vi "Dashboard Main.vi"() -> ()   [LabVIEW 2017]
uses:
  <vilib>/Utility/miscctls.llb/LVRowAndColumnTypeDef.ctl
  <vilib>/event_ctls.llb/eventvkey.ctl
  <vilib>/Rock Robotics/Network Tables/NT Read Numeric Array.vi
  <vilib>/Rock Robotics/Network Tables/NT Read Boolean.vi
  <vilib>/Rock Robotics/WPI/Dashboard/WPI_DashboardLogging Global.vi
panel:
  in  "Camera Settings Right":T1={"Frame Rate"=30, "Compression"=30, "Size"=1, "DB Camera Config"=FALSE} {"Frame Rate" scale=1.0..30.0; "Compression" scale=100.0..-1.0; "Size" items=["640x480", "320x240", "160x120"]}
  in  "Camera Name Right":string(combo)="No Camera Selection"
  out "Camera Info":cluster{"Mbps LED":bool, "Mbps":dbl, "fps":dbl} {"fps" format="%#.1g"; "Mbps" format="%#.1g"}
  in  "Camera Settings":T1={"Frame Rate"=30, "Compression"=30, "Size"=1, "DB Camera Config"=FALSE} {"Frame Rate" scale=1.0..30.0; "Compression" scale=100.0..-1.0; "Size" items=["640x480", "320x240", "160x120"]}
  in  "TCP":refnum<k5>
  in  "Rec Mode":enum32{"Stop", "Record", "Playback"}(radio)
  out "Robot IP":string
  out "Image Message":string="Timeout in Camera Communications"
  in  "Dashboard Tab":T2(tab)
  in  "Select Auto":string(combo)="Select Autonomous ..."
  out "NT Connection":bool
  out "MotorChart R":cluster{"Numeric":dbl, "Numeric":dbl}(graph)
  out "MotorChart L":cluster{"Numeric":dbl, "Numeric":dbl}(graph)
  out "MotorSliders R":cluster{"MotorSlide1":dbl, "MotorSlide2":dbl} {"MotorSlide2" scale=-1.0..1.0 scale format="%#_2e"; "MotorSlide1" scale=-1.0..1.0 scale format="%#_2e"}
  out "MotorSliders L":cluster{"MotorSlide1":dbl, "MotorSlide2":dbl} {"MotorSlide2" scale=-1.0..1.0 scale format="%#_2e"; "MotorSlide1" scale=-1.0..1.0 scale format="%#_2e"}
  out "Gyro":dbl(knob) scale=0.0..360.0
  out "JS1 Z":dbl(slide) scale=-1.0..1.0 scale format="%#_2e"
  out "JS1 Graph":cluster{"X":dbl, "Y":dbl}[](graph)
  out "JS1 Buttons":T3
  out "JS2 Z":dbl(slide) scale=-1.0..1.0 scale format="%#_2e"
  out "JS2 Graph":cluster{"X":dbl, "Y":dbl}[](graph)
  out "JS2 Buttons":T3
  out "Mode":T4(ring)=enum."Auto Disabled"
  out "Camera Image Right":T5(plugin-control)
  in  "DB/String 9":string
  in  "DB/String 8":string
  in  "DB/String 7":string
  in  "DB/String 6":string
  in  "DB/String 5":string
  in  "DB/String 4":string
  in  "DB/String 3":string
  in  "DB/String 2":string
  in  "DB/String 1":string
  in  "DB/String 0":string
  in  "DB/Slider 0":dbl(slide) scale=0.0..5.0
  in  "DB/Slider 1":dbl(slide) scale=0.0..5.0
  in  "DB/Slider 2":dbl(slide) scale=0.0..5.0
  in  "DB/Slider 3":dbl(slide) scale=0.0..5.0
  out "DB/LED 3":bool
  out "DB/LED 2":bool
  out "DB/LED 1":bool
  out "DB/LED 0":bool
  in  "DB/Button 3":bool
  in  "DB/Button 2":bool
  in  "DB/Button 1":bool
  in  "DB/Button 0":bool caption="New Name"
  in  "Derrivative 2":dbl
  in  "Proportion 2":dbl
  in  "Integral 2":dbl
  in  "Derrivative":dbl
  in  "Integral":dbl
  in  "Proportion":dbl
  out "Lower Limit":bool
  out "Upper Limit":bool
  in  "Encoder distance":dbl
  in  "Test Slider":dbl(slide) scale=0.0..100.0 scale format="%#_3g"
  in  "On/Off":bool caption="Solenoid"
  in  "Test Name":u16(ring) items=["Select the test to run..."]
  in  "Test Tree":string(tree)
  in  "Motor":cluster{"Value":dbl, "Enable":bool} {"Value" scale=-1.0..1.0 scale format="%#_3g"}
  out "Progress":T6 {"Test Progress" scale=0.0..100.0}
  in  "Rev/Fwd":cluster{"Forward":bool, "Reverse":bool}
  in  "Test Ring":u16(ring) items=["Monochrome", "Color"]
  out "Cmd Status":string
  in  "Execute Command":bool
  in  "Command Params":string[][](table)
  in  "Command Selection":i32(listbox)
  in  "CheckList":i32(listbox)
  out "Tree":string(tree)
  out "Camera Image":T5(plugin-control)
  out "Background":bool
  in  "Camera Name":string(combo)="No Camera Selection"
  # "HW"
  # "HW"
  # "Joysticks"
  # "Drive Motors"
  # "Front"
  # "Right"
  # "Left"
  # "Back"
  # "Left Drive"
  # "Right (Follow)  Drive"
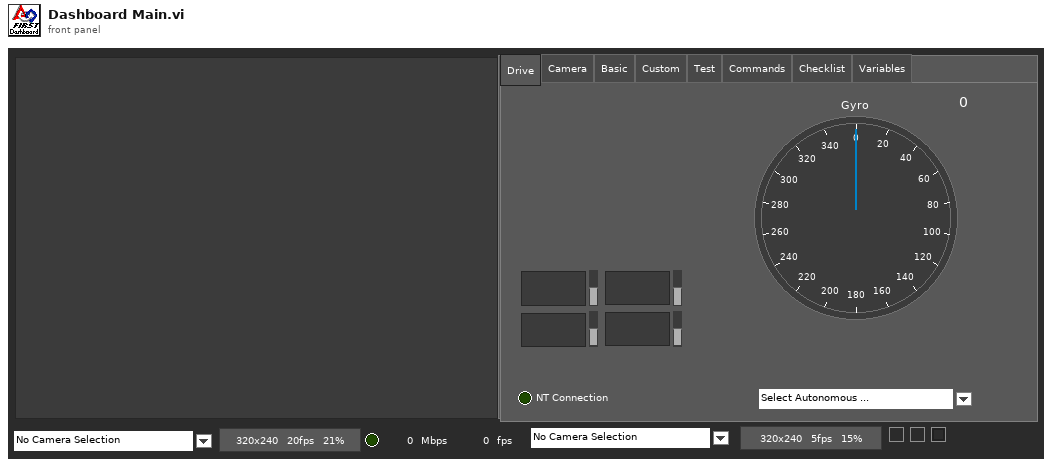
[diagram p1: front panel]
types:
  T1 = cluster{"Frame Rate":i32, "Compression":i32, "Size":u16, "DB Camera Config":bool}
  T2 = enum32{"Drive", "Camera", "Basic", "Custom", "Test", "Commands", "Checklist", "Variables"}
  T3 = cluster{bool, bool, bool, bool, bool, bool, bool, bool, bool, bool, bool, bool}
  T4 = enum8{"Tele-Op Disabled", "Tele-Op Enabled", "Auto Disabled", "Auto Enabled", "Test Disabled", "Test Enabled", "Disconnected", "No Code", "E-Stop"}
  T5 = typedef "IMAQ Image.ctl" = refnum<image>
  T6 = cluster{"Test Progress":u8, "Test Progress Text":string}
  T7 = cluster{"Save Path":path, "Interval (s)":dbl, "Keep":i32}
  T8 = typedef "Image Type" = u32
  T9 = cluster{"IDs":cluster{"RPC field ID":u16, "Unique ID":u16}, "String":string}
  T10 = cluster{"Error Strings":string, "Disable Counts":cluster{u16, u16}, "Rail Faults":cluster{u16, u16, u16}, "Robot IP":string, "DB Mode":u8, "Event Info":cluster{"Name":string, "Type":u8, "Number":u16, "Replay":u8}}
  T11 = cluster{"Storage":cluster{"Disk Free":u64, "RAM Block":u32, "RAM free":u32}, "CPU Utilization":cluster{"CPU % ISR":sgl, "CPU % Time Crit":sgl, "CPU % Timed Str":sgl, "CPU % High":sgl, "CPU % Above":sgl, "CPU % Normal":sgl, "CPU % Low":sgl}, "CAN":cluster{"% Bus Utilization":sgl, "Bus Off Cnt":u32, "TX_FIFO Full Cnt":u32, "Receive Error Cnt":u8, "Transmit Error Cnt":u8}, "HID":cluster{"HID Outputs":u32, "Rumble Low":u16, "Rumble High":u16}[]}
  T12 = cluster{"Status bits":cluster{"Test Mode":bool, "Autonomous":bool, "Enabled":bool, "Code Start":bool, "Brownout":bool, "Reserved 2":bool, "Reserved 3":bool, "E-Stop":bool}, "Code Trace":cluster{"Disabled":bool, "TeleOp":bool, "Auto":bool, "Test":bool}, "Controller Type":enum16{"unknown", "cRIO", "roboRio"}, "Code?":enum16{"unknown", "noCode", "code"}, "Battery V":dbl}
  T13 = cluster{"Control Bits":cluster{"TestMode":bool, "Autonomous":bool, "Enabled":bool, "FMS Present":bool, bool, bool, bool, "E-Stop":bool}, "Team Station ":u8, "Countdown":sgl, "Joystick Values":cluster{"Axes":dbl[], "Buttons":bool[], "POVs":i16[]}[]}
  T14 = cluster{"Axes":dbl[], "Buttons":bool[], "POVs":i16[]}[]
  T15 = cluster{"Axes":dbl[], "Buttons":bool[], "POVs":i16[]}
  T16 = cluster{"Buttons[0]":bool, "Buttons[1]":bool, "Buttons[2]":bool, "Buttons[3]":bool, "Buttons[4]":bool, "Buttons[5]":bool, "Buttons[6]":bool, "Buttons[7]":bool, "Buttons[8]":bool, "Buttons[9]":bool, "Buttons[10]":bool, "Buttons[11]":bool}
  T17 = cluster{"Camera Image":refnum<vi>, "Dashboard Tab":refnum<vi>, "Background":refnum<vi>, "Rec Mode":refnum<vi>, "Test Slider":refnum<vi>, "On/Off ":refnum<vi>, "Test Ring":refnum<vi>, "Rev/Fwd":refnum<vi>, "Test Name":refnum<vi>, "Motor":refnum<vi>, "Progress":refnum<vi>, "CheckList":refnum<vi>, "Tree":refnum<vi>, "Test Tree":refnum<vi>, "Command Params":refnum<vi>, "Command Selection":refnum<vi>, "Execute Command":refnum<vi>, "Cmd Status":refnum<vi>, "Camera Settings":refnum<vi>, "Camera Name":refnum<vi>, "Camera Info":refnum<vi>, "Camera Settings Right":refnum<vi>, "Camera Name Right":refnum<vi>, "Camera Image Right":refnum<vi>}
  T18 = cluster{"Camera Name":string, string, "Saved DB Images Info":cluster{"Save Path":path, "Interval (s)":dbl, "Keep":i32}}
  T19 = cluster{"Camera Name Right":string, string, "Saved DB Images Info":cluster{"Save Path":path, "Interval (s)":dbl, "Keep":i32}}
  T20 = cluster{"Operation":enum16{"Update", "Clear"}, "Color Box":u32}[]
  T21 = typedef "eventvkey.ctl" = enum16{"ASCII", "Enter", "Return", "Shift", "Ctrl", "Alt", "Cmd", "Opt", "Caps", "NumLock", "Clear", "Break", "Up", "Down", "Left", "Right", "Insert", "Delete", "Home", "End", "PageUp", "PageDown", "Escape", "Help", "Pause", "ScrollLock", "F1", "F2", "F3", "F4", "F5", "F6", "F7", "F8", "F9", "F10", "F11", "F12", "F13", "F14", "F15", "F16", "F17", "F18", "F19", "F20", "F21", "F22", "F23", "F24", "Play", "VolumeUp", "VolumeDown", "Mute", "Two Byte Char"}
  T22 = cluster{"Image Size":bool, "Image Type":bool, "Pixel Value":bool, "ROI Information":bool, "Zoom Factor":bool}
  T23 = cluster{"Operation":enum16{"Update", "Clear"}, "Color Box":u32}
  T24 = typedef "LVRowAndColumnTypeDef.ctl" = cluster{"Row":i32, "Column":i32}
  T25 = cluster{"Shift":bool, "Ctrl":bool, "Alt":bool, "Cmd":bool, "Opt":bool}
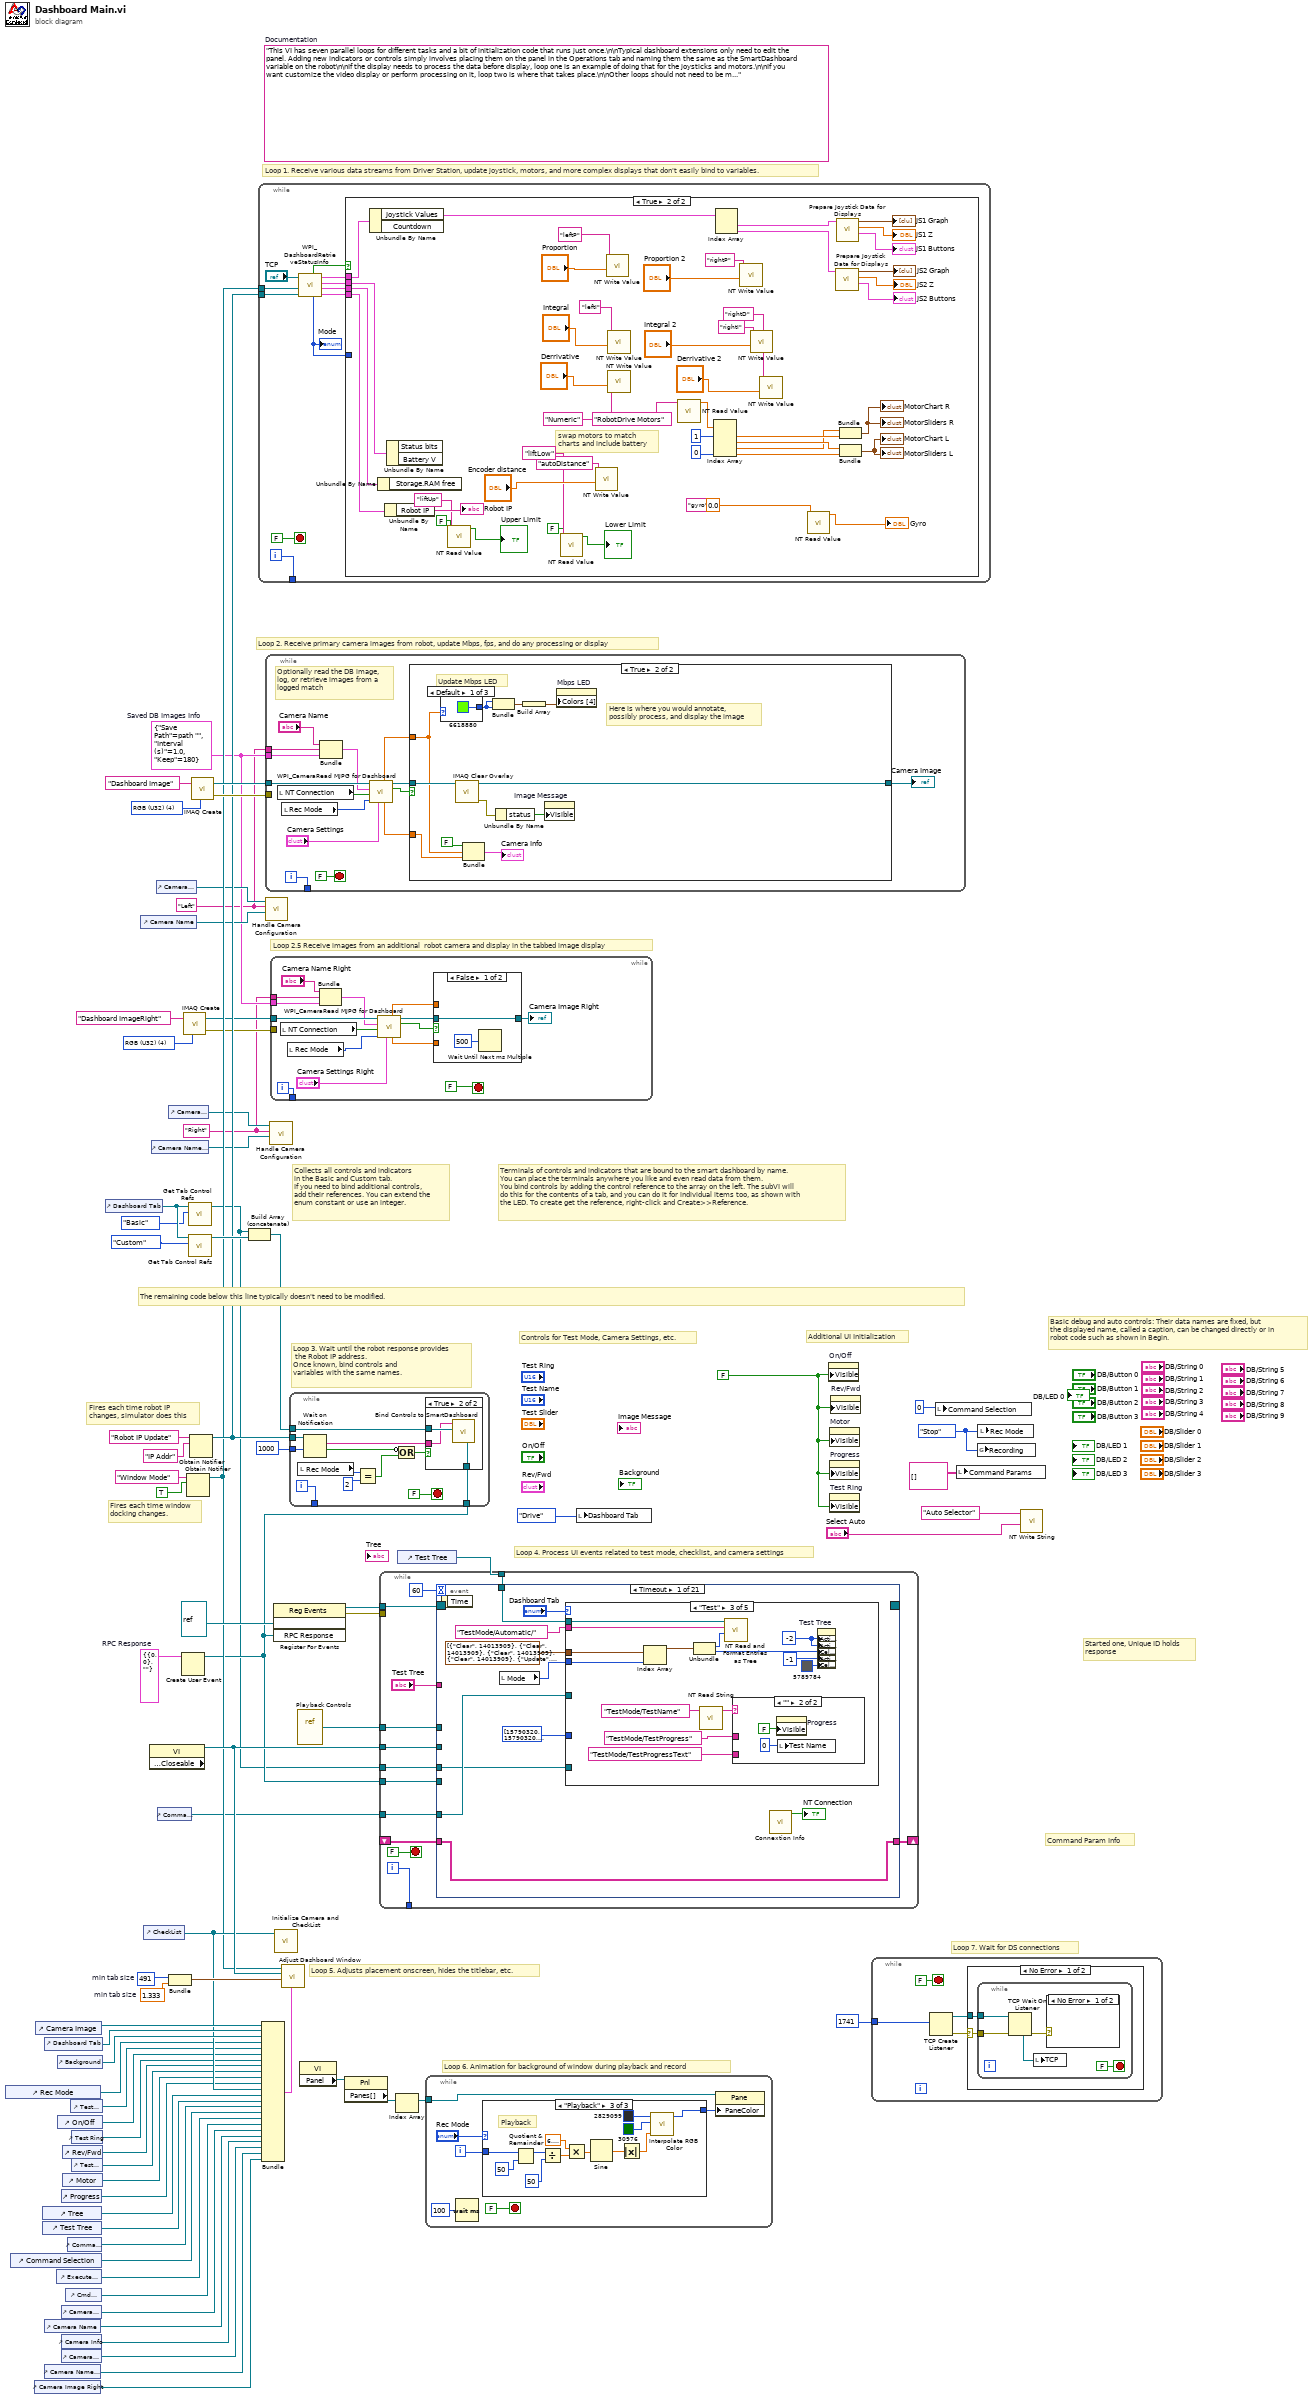
[diagram p0: block diagram]
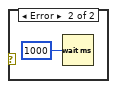
[diagram p3: hidden frame]
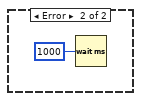
[diagram p4: hidden frame]
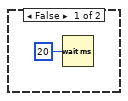
[diagram p5: hidden frame]
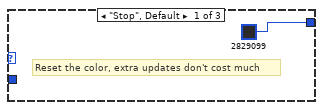
[diagram p6: hidden frame]
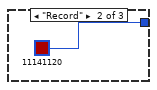
[diagram p7: hidden frame]
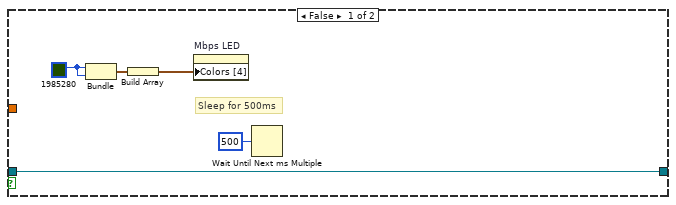
[diagram p9: hidden frame]
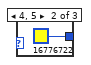
[diagram p10: hidden frame]
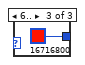
[diagram p11: hidden frame]
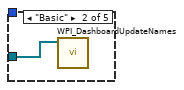
[diagram p13: hidden frame]
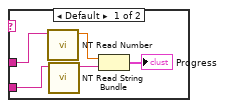
[diagram p14: hidden frame]
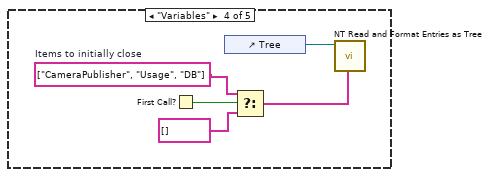
[diagram p15: hidden frame]
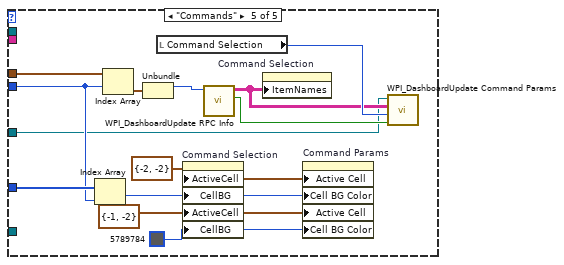
[diagram p16: hidden frame]
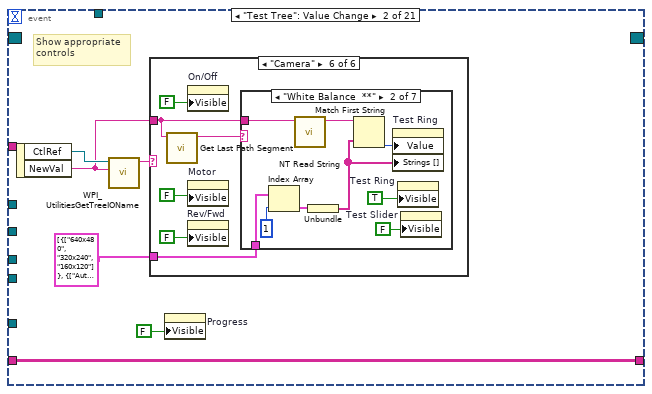
[diagram p17: hidden frame]
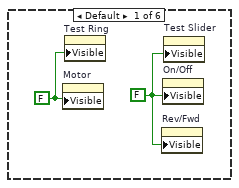
[diagram p18: hidden frame]
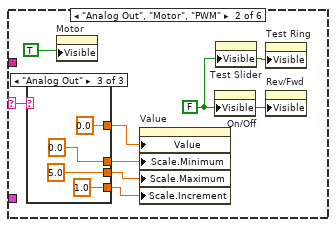
[diagram p19: hidden frame]
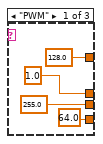
[diagram p20: hidden frame]
diagram:
  w3 = T7 {"Save Path"=path "", "Interval (s)"=1.0, "Keep"=180}  # Saved DB Images Info
  w2 = "Right"
  w1 = "Left"
  w13 = T8 4 items=["Grayscale (U8)", "Grayscale (I16)", "Grayscale (SGL)", "Complex (CSG)", "RGB (U32)", "HSL (U32)", "RGB (U64)"] ("Image Type")
  w29 = T9 {"IDs"={"RPC field ID"=0, "Unique ID"=0}, "String"=""}  # RPC Response
  w52 = 491  # min tab size
  w51 = 1.333  # min tab size
  w59 = enum32{"Stop", "Record", "Playback"}."Stop" ("Rec Mode")
  w36 = FALSE ("Visible")
  (unwired) "This VI has seven parallel loops for different tasks and a bit of initialization code that runs just once.\n\nTypical dashboard extensions only need to edit the panel. Adding new indicators or controls simply involves placing them on the panel in the Operations tab and naming them the same as the SmartDashboard variable on the robot\n\nIf the display needs to process the data before display, loop one is an example of doing that for the joysticks and motors.\n\nIf you want customize the video display or perform processing on it, loop two is where that takes place.\n\nOther loops should not need to be modified. They are pretty standard, and document the task they perform."  # Documentation
  w76 = T8 4 items=["Grayscale (U8)", "Grayscale (I16)", "Grayscale (SGL)", "Complex (CSG)", "RGB (U32)", "HSL (U32)", "RGB (U64)"] ("Image Type")
  # "Loop 2.5 Receive images from an additional  robot camera and display in the tabbed image display"
  # "Command Param Info"
  # "Started one, Unique ID holds\nresponse"
  # "Loop 7. Wait for DS connections"
  # "Basic debug and auto controls: Their data names are fixed, but\nthe displayed name, called a caption, can be changed directly or in\nrobot code such as shown in Begin."
  # "Controls for Test Mode, Camera Settings, etc."
  # "Additional UI Initialization"
  # "Loop 6. Animation for background of window during playback and record"
  # "Fires each time robot IP\nchanges, simulator does this"
  # "Fires each time window\ndocking changes."
  # "Collects all controls and indicators\nin the Basic and Custom tab.\nIf you need to bind additional controls,\nadd their references. You can extend the\nenum constant or use an integer."
  # "The remaining code below this line typically doesn't need to be modified."
  # "Loop 4. Process UI events related to test mode, checklist, and camera settings"
  # "Terminals of controls and indicators that are bound to the smart dashboard by name.\nYou can place the terminals anywhere you like and even read data from them.\nYou bind controls by adding the control reference to the array on the left. The subVI will\ndo this for the contents of a tab, and you can do it for individual items too, as shown with\nthe LED. To create get the reference, right-click and Create>>Reference."
  # "Loop 3. Wait until the robot response provides\n the Robot IP address.\nOnce known, bind controls and\nvariables with the same names."
  # "Loop 5. Adjusts placement onscreen, hides the titlebar, etc."
  # "Loop 1. Receive various data streams from Driver Station, update joystick, motors, and more complex displays that don't easily bind to variables."
  # "Loop 2. Receive primary camera images from robot, update Mbps, fps, and do any processing or display"
  n1 = control-ref of="Rec Mode"() -> (w42:refnum<vi>)
  n2 = control-ref of="Command Selection"() -> (w28:refnum<vi>)
  n3 = control-ref of="Camera Image Right"() -> (w6:refnum<vi>)
  n4 = control-ref of="Camera Image"() -> (w54:refnum<vi>)
  n5 = control-ref of="Tree"() -> (w46:refnum<vi>)
  n6 = control-ref of="Test Tree"() -> (w45:refnum<vi>)
  n7 = control-ref of="Dashboard Tab"() -> (w53:refnum<vi>)
  n8 = control-ref of="Camera Name"() -> (w19:refnum<vi>)
  n9 = control-ref of="Camera Name Right"() -> (w7:refnum<vi>)
  n10 = control-ref of="Execute Command"() -> (w30:refnum<vi>)
  n11 = control-ref of="Background"() -> (w49:refnum<vi>)
  n12 = control-ref of="On/Off"() -> (w40:refnum<vi>)
  n13 = control-ref of="Progress"() -> (w37:refnum<vi>)
  n14 = control-ref of="Camera Settings"() -> (w20:refnum<vi>)
  n15 = control-ref of="Camera Info"() -> (w18:refnum<vi>)
  n16 = control-ref of="Camera Settings Right"() -> (w8:refnum<vi>)
  n17 = control-ref of="Rev/Fwd"() -> (w38:refnum<vi>)
  n18 = control-ref of="Motor"() -> (w43:refnum<vi>)
  n19 = control-ref of="Cmd Status"() -> (w24:refnum<vi>)
  n20 = control-ref of="Command Params"() -> (w31:refnum<vi>)
  n21 = control-ref of="Test Slider"() -> (w41:refnum<vi>)
  n22 = control-ref of="Test Ring"() -> (w39:refnum<vi>)
  n23 = control-ref of="Test Name"() -> (w44:refnum<vi>)
  n24 = control-ref of="Dashboard Tab"() -> (w57:refnum<vi>)
  n25 = control-ref of="Camera Name"() -> (w21:refnum<vi>)
  n26 = control-ref of="CheckList"() -> (w47:refnum<vi>)
  n27 = property class="VI" props=["Front Panel.Closeable"]() -> (reference out=w58:refnum<vi>)  [unwired: 2 in, 2 out]
  n28 = control-ref of="Camera Name Right"() -> (w9:refnum<vi>)
  n29 = control-ref of="Camera Settings"() -> (w22:refnum<vi>)
  n30 = control-ref of="Command Params"() -> (w23:refnum<vi>)
  n31 = control-ref of="Camera Settings Right"() -> (w10:refnum<vi>)
  n32 = Bundle("min tab size"=w52, "min tab size"=w51) -> (w50:cluster{"min tab size":i32, "min tab size":dbl})  [unwired: 1 in]
  n33 = Create User Event(user event datatype=w29) -> (user event=w25:refnum<user-event>)  [unwired: 1 in, 1 out]
  n34 = call "IMAQ Create"("Image Name"="Dashboard ImageRight", "Image Type"=w13) -> ("New Image"=w12:T5, "error out"=w11:errorcluster)  [unwired: 2 in, 1 out]
  n35 = Obtain Notifier(name (unnamed)="Window Mode", notification data type=TRUE) -> (notifier out=w34:refnum<notifier>)  [unwired: 2 in, 2 out]
  n36 = call <vilib>:"Get Tab Control Refs.vi"("Page Index"=T2."Basic" ("Dashboard Tab"), "TabControl in"=w57) -> ("ControlsOnPage"=w17:refnum<vi>[])  [unwired: 9 in]
  n37 = call <vilib>:"Get Tab Control Refs.vi"("Page Index"=T2."Custom" ("Dashboard Tab"), "TabControl in"=w57) -> ("ControlsOnPage"=w56:refnum<vi>[])  [unwired: 9 in]
  n38 = Obtain Notifier(name (unnamed)="Robot IP Update", notification data type="IP Addr" ("name (unnamed)")) -> (notifier out=w35:refnum<notifier>)  [unwired: 2 in, 2 out]
  n39 = call "IMAQ Create"("Image Name"="Dashboard Image", "Image Type"=w76) -> ("New Image"=w74:T5, "error out"=w73:errorcluster)  [unwired: 2 in, 1 out]
  n40 = Build Array (concatenate)(w17, w56) -> (w55:refnum<vi>[])
  n41 = while {
    tunnel: [w86] -> _
    tunnel: w35 -> [w80]
    tunnel: w34 -> [w77]
    i -> [w86]
    stop <- FALSE stop-if-true
    n42 = call <vilib>:"WPI_DashboardRetrieveStatusInfo.vi"("Binding Refnum"=w80, "Window Mode Notifier"=w77, "TCP Cnx"="TCP") -> ("Power and Errors"=w81:T10, "Robot Metrics"=w84:T11, "Status Info"=w85:T12, "Control Info"=w82:T13, "Robot Mode"=w79:T4, "Process?"=w83:bool)  [unwired: 3 in]
    "Mode" <- w79
    n43 = case shown="True" w83 {
      tunnel: w85 -> [_ w135]
      tunnel: w84 -> [_ w134]
      tunnel: w82 -> [_ w133]
      tunnel: w81 -> [_ w132]
      tunnel: w79 -> [_ _]
      frame False {
        n44 = Wait (ms)(milliseconds to wait=u32 20) -> ()  [unwired: 1 out]
      }
      frame True {
        # "swap motors to match\ncharts and include battery"
        n45 = Unbundle By Name(w133) -> ("Joystick Values"=w123:T14)  [unwired: 1 out]
        n46 = Unbundle By Name(w134) -> ()  [unwired: 1 out]
        n47 = Unbundle By Name(w132) -> ("Robot IP"=→"Robot IP":string)
        n48 = Unbundle By Name(w135) -> ()  [unwired: 2 out]
        n49 = call-poly <vilib>:"NT Read Value.vi"("Default Value"=FALSE, "Name"="liftUp") -> ("Boolean"=→"Upper Limit":bool)  [unwired: 8 in, 1 out]
        n50 = call-poly <vilib>:"NT Read Value.vi"("Default Value"=FALSE, "Name"="liftLow") -> ("Boolean"=→"Lower Limit":bool)  [unwired: 8 in, 1 out]
        n51 = call-poly <vilib>:"NT Write Value.vi"("Numeric"="Encoder distance", "Name"="autoDistance") -> ()  [unwired: 9 in, 1 out]
        n52 = call-poly <vilib>:"NT Write Value.vi"("Numeric"="Proportion", "Name"="leftP") -> ()  [unwired: 9 in, 1 out]
        n53 = call-poly <vilib>:"NT Write Value.vi"("Numeric"="Integral", "Name"="leftI") -> ()  [unwired: 9 in, 1 out]
        n54 = call-poly <vilib>:"NT Write Value.vi"("Numeric"="Derrivative", "Name"="Numeric") -> ()  [unwired: 9 in, 1 out]
        n55 = call-poly <vilib>:"NT Read Value.vi"("Name"="RobotDrive Motors") -> ("Numeric Array"=w113:dbl[])  [unwired: 9 in, 1 out]
        n56 = Index Array(array=w113, index #1=1, index #4=0) -> (element #1=w127:dbl, element #2=w128:dbl, element #3=w126:dbl, element #4=w131:dbl)  [unwired: 2 in]
        n57 = Index Array(array=w123) -> (element #1=w122:T15, element #2=w118:T15)  [unwired: 2 in]
        n58 = call-poly <vilib>:"NT Write Value.vi"("Numeric"="Proportion 2", "Name"="rightP") -> ()  [unwired: 9 in, 1 out]
        n59 = call-poly <vilib>:"NT Write Value.vi"("Numeric"="Integral 2", "Name"="rightI") -> ()  [unwired: 9 in, 1 out]
        n60 = call-poly <vilib>:"NT Write Value.vi"("Numeric"="Derrivative 2", "Name"="rightD") -> ()  [unwired: 9 in, 1 out]
        n61 = call-poly <vilib>:"NT Read Value.vi"("Default Value"=0.0, "Name"="gyro") -> ("Numeric"=→"Gyro":dbl)  [unwired: 8 in, 1 out]
        n62 = call "Prepare Joystick Data for Displays.vi"("Joystick Values"=w118) -> ("Buttons"=→"JS2 Buttons":T16, "Z Axis"=→"JS2 Z":dbl, "Cartesian Data"=→"JS2 Graph":cluster{"X axis":dbl, "X axis":dbl}[])  [unwired: 8 in]
        n63 = call "Prepare Joystick Data for Displays.vi"("Joystick Values"=w122) -> ("Buttons"=→"JS1 Buttons":T16, "Z Axis"=→"JS1 Z":dbl, "Cartesian Data"=→"JS1 Graph":cluster{"X axis":dbl, "X axis":dbl}[])  [unwired: 8 in]
        n64 = Bundle("Numeric"=w126, "Numeric"=w127) -> (→"MotorChart R" →"MotorSliders R":cluster{"Numeric":dbl, "Numeric":dbl})  [unwired: 1 in]
        n65 = Bundle("Numeric"=w128, "Numeric"=w131) -> (→"MotorChart L" →"MotorSliders L":cluster{"Numeric":dbl, "Numeric":dbl})  [unwired: 1 in]
      }
    }
  }
  n66 = Bundle("Camera Image"=w54, "Dashboard Tab"=w53, "Background"=w49, "Rec Mode"=w42, "Test Slider"=w41, "On/Off"=w40, "Test Ring"=w39, "Rev/Fwd"=w38, "Test Name"=w44, "Motor"=w43, "Progress"=w37, "CheckList"=w47, "Tree"=w46, "Test Tree"=w45, "Command Params"=w31, "Command Selection"=w28, "Execute Command"=w30, "Cmd Status"=w24, "Camera Settings"=w20, "Camera Name"=w19, "Camera Info"=w18, "Camera Settings Right"=w8, "Camera Name Right"=w7, "Camera Image Right"=w6) -> (w48:T17)  [unwired: 1 in]
  n67 = call "Handle Camera Configuration.vi"("CameraNameRef"=w21, "Display Name"=w1, "ClusterRef"=w22) -> ()  [unwired: 9 in]
  n68 = while {
    tunnel: w74 -> [w148]
    tunnel: w73 -> [_]
    tunnel: [w149] -> _
    tunnel: w3 -> [w139]
    tunnel: w1 -> [w136]
    i -> [w149]
    stop <- FALSE stop-if-true
    # "Optionally read the DB image,\nlog, or retrieve images from a\nlogged match"
    n69 = local read "NT Connection"() -> (w140:bool)
    n70 = local read "Rec Mode"() -> (w144:enum32{"Stop", "Record", "Playback"})
    n71 = Bundle("Camera Name"="Camera Name", w136, "Saved DB Images Info"=w139) -> (w138:T18)  [unwired: 1 in]
    n72 = call <vilib>:"WPI_CameraRead MJPG for Dashboard.vi"("Camera Settings"="Camera Settings", "Rec Mode"=w144, "NT Connection"=w140, "Capture Info"=w138, "Refnum in"=w148) -> ("Active"=w146:bool, "Refnum out"=w147:T5, "FPS"=w145:dbl, "Bandwidth (Mbps)"=w143:dbl)  [unwired: 3 in]
    n73 = case shown="True" w146 {
      tunnel: w147 -> [w151 w162]
      tunnel: w143 -> [_ w159]
      tunnel: w145 -> [_ w160]
      tunnel: [w151 w156] -> w141
      frame False {
        w153 = u32 1985280 ("Color Box")
        # "Sleep for 500ms"
        n74 = Bundle("Color Box"=w153, "Color Box"=w153) -> (w154:cluster{"Color Box":u32, "Color Box":u32})  [unwired: 1 out]
        n75 = Build Array(w154) -> (w152:cluster{"Color Box":u32, "Color Box":u32}[])
        n76 = property on="Mbps LED" class="Bool (strict)"("Colors [4]"=w152) -> ()  [unwired: 2 in, 2 out]
        n77 = Wait Until Next ms Multiple(millisecond multiple=u32 500) -> ()  [unwired: 1 out]
      }
      frame True {
        # "Here is where you would annotate,\npossibly process, and display the image"
        # "Update Mbps LED"
        n78 = case shown="Default" w159 {
          tunnel: [u32 6618880 ("Color Box") u32 16776722 ("Color Box") u32 16716800 ("Color Box")] -> w163
          frame Default {
          }
          frame 4, 5 {
          }
          frame 6.. {
          }
        }
        n79 = call "IMAQ Clear Overlay"("Image"=w162) -> ("error out"=w165:errorcluster, "Image Out"=w156:T5)  [unwired: 2 in, 7 out]
        n80 = Bundle(FALSE, "Bandwidth (Mbps)"=w159, "FPS"=w160) -> (→"Camera Info":cluster{bool, "Bandwidth (Mbps)":dbl, "FPS":dbl})  [unwired: 1 in]
        n81 = Bundle("Color Box"=w163, "Color Box"=w163) -> (w164:cluster{"Color Box":u32, "Color Box":u32})  [unwired: 1 out]
        n82 = Unbundle By Name(w165) -> ("status"=w166:bool)
        n83 = Build Array(w164) -> (w161:cluster{"Color Box":u32, "Color Box":u32}[])
        n84 = property on="Image Message" class="Str"("Visible"=w166) -> ()  [unwired: 2 in, 2 out]
        n85 = property on="Mbps LED" class="Bool (strict)"("Colors [4]"=w161) -> ()  [unwired: 2 in, 2 out]
      }
    }
    "Camera Image" <- w141
  }
  n86 = call "Handle Camera Configuration.vi"("CameraNameRef"=w9, "Display Name"=w2, "ClusterRef"=w10) -> ()  [unwired: 9 in]
  n87 = while {
    tunnel: w12 -> [w184]
    tunnel: w11 -> [_]
    tunnel: [w179] -> _
    tunnel: w3 -> [w173]
    tunnel: w2 -> [w170]
    i -> [w179]
    stop <- FALSE stop-if-true
    n88 = local read "NT Connection"() -> (w174:bool)
    n89 = local read "Rec Mode"() -> (w183:enum32{"Stop", "Record", "Playback"})
    n90 = Bundle("Camera Name Right"="Camera Name Right", w170, "Saved DB Images Info"=w173) -> (w172:T19)  [unwired: 1 in]
    n91 = call <vilib>:"WPI_CameraRead MJPG for Dashboard.vi"("Camera Settings"="Camera Settings Right", "Rec Mode"=w183, "NT Connection"=w174, "Capture Info"=w172, "Refnum in"=w184) -> ("Active"=w178:bool, "Refnum out"=w181:T5, "FPS"=w176:dbl, "Bandwidth (Mbps)"=w177:dbl)  [unwired: 3 in]
    n92 = case shown="False" w178 {
      tunnel: w181 -> [w185 w187]
      tunnel: w177 -> [_ _]
      tunnel: w176 -> [_ _]
      tunnel: [w185 w187] -> w175
      frame False {
        n93 = Wait Until Next ms Multiple(millisecond multiple=u32 500) -> ()  [unwired: 1 out]
      }
      frame True {
      }
    }
    "Camera Image Right" <- w175
  }
  n94 = register-events(refnum<vi> refnum, w25) -> (reference out=w63:refnum<event-registration>, error out=w62:errorcluster)  [unwired: 2 in]
  n95 = call "Initialize Camera and CheckList.vi"("ListBox in"=w47) -> ()  [unwired: 11 in]
  n96 = call "Adjust Dashboard Window.vi"("Sizing Refnums"=w48, "Size Constraints"=w50, "VI"=w58, "WIn Mode"=w34) -> ()  [unwired: 8 in]
  n97 = while {
    tunnel: w55 -> [w199]
    tunnel: w35 -> [w197]
    tunnel: [w195] -> _
    tunnel: u32 1000 ("milliseconds to wait") -> [w194]
    tunnel: w25 -> [w188]
    i -> [w195]
    stop <- FALSE stop-if-true
    n98 = local read "Rec Mode"() -> (w190:enum32{"Stop", "Record", "Playback"})
    n99 = Wait on Notification(notifier=w197, timeout in ms (-1)=w194) -> (notification=w196:string, timed out?=w192:bool)  [unwired: 2 in, 2 out]
    n100 = Equal?(x=w190, y=u16 2 ("Rec Mode")) -> (x = y?=w191:bool)
    n101 = Compound Arithmetic op=OR(invert w192, w191) -> (w193:bool)
    n102 = case shown="True" w193 {
      tunnel: w199 -> [_ w202]
      tunnel: w196 -> [_ w201]
      tunnel: w188 -> [_ w200]
      frame False {
      }
      frame True {
        n103 = call <vilib>:"Bind Controls to SmartDashboard.vi"("RPC ref"=w200, "Bound Control Refs"=w202, "Server IP Address"=w201) -> ()  [unwired: 9 in]
      }
    }
  }
  n104 = vi-ref "Playback Controls.vi"() -> (w64:refnum<vi>)
  n105 = property class="VI"() -> ("Panel"=w66:refnum<vi>)  [unwired: 2 in, 2 out]
  n106 = property class="Pnl"(reference=w66) -> ("Panes[]"=w67:refnum<vi>[])  [unwired: 1 in, 2 out]
  n107 = Index Array(array=w67) -> (element=w65:refnum<vi>)  [unwired: 1 in]
  n108 = control-ref of="Test Tree"() -> (w68:refnum<vi>)
  n109 = while {
    tunnel: [w212] -> _
    tunnel: w68 -> [w211]
    tunnel: w64 -> [w210]
    tunnel: w63 -> [w209]
    tunnel: w62 -> [_]
    tunnel: w58 -> [w208]
    tunnel: w25 -> [w207]
    tunnel: w23 -> [w206]
    shift-right: [w205] -> _
    shift-left: _ -> [w204]
    tunnel: w17 -> [w203]
    i -> [w212]
    stop <- FALSE stop-if-true
    n110 = event shown="[0] Timeout" {
      selector: w209 -> [_ _ _ _ _ _ _ _ _ _ _ _ _ _ _ _ _ _ _ _ _]
      dyn-events: [_ _ _ _ _ _ _ _ _ _ _ _ _ _ _ _ w472 _ _ _ _] -> _
      timeout: u32 60 ("milliseconds to wait") -> [_ _ _ _ _ _ _ _ _ _ _ _ _ _ _ _ _ _ _ _ _]
      tunnel: w211 -> [w224 _ _ _ _ _ _ _ _ _ _ _ _ _ _ _ _ _ _ _ _]
      tunnel: "Test Tree" -> [_ _ _ _ _ _ _ _ _ _ _ w439 w447 w449 w453 w461 _ _ _ _ _]
      tunnel: w210 -> [_ _ _ _ _ _ _ _ _ _ _ _ _ _ _ _ w474 _ w492 _ _]
      tunnel: w208 -> [_ _ _ _ _ _ _ _ _ _ _ _ _ _ _ _ w470 _ _ _ _]
      tunnel: w207 -> [_ _ _ _ _ _ _ _ _ _ _ _ _ _ _ _ w468 _ _ _ _]
      tunnel: w206 -> [w219 _ _ _ _ _ w390 _ _ _ _ _ _ _ _ _ _ _ _ _ _]
      tunnel: [w218 w267 w369 w374 w383 w387 w388 w397 w407 w414 w426 w438 w445 w448 w452 w460 w467 w487 w489 w493 w506] -> w205
      tunnel: w204 -> [w218 w267 w369 w374 w383 w387 w388 _ _ w414 w426 w438 w445 w448 w452 w460 w467 w487 w489 w493 w506]
      tunnel: w203 -> [w216 _ _ _ _ _ _ _ _ _ _ _ _ _ _ _ _ _ _ _ _]
      event Timeout {
        n111 = event-data() -> ()  [unwired: 1 in, 1 out]
        n112 = local read "Mode"() -> (w221:T4)
        n113 = case shown="\"Test\"" "Dashboard Tab" {
          tunnel: w224 -> [_ _ w240 _ _]
          tunnel: "TestMode/Automatic/" ("Name Pattern") -> [_ _ w239 _ _]
          tunnel: T20 [{"Operation"=enum."Clear", "Color Box"=14013909}, {"Operation"=enum."Clear", "Color Box"=14013909}, {"Operation"=enum."Clear", "Color Box"=14013909}, {"Operation"=enum."Clear", "Color Box"=14013909}, {"Operation"=enum."Update", "Color Box"=14013909}, {"Operation"=enum."Update", "Color Box"=16777215}, {"Operation"=enum."Clear", "Color Box"=14013909}, {"Operation"=enum."Clear", "Color Box"=14013909}, {"Operation"=enum."Clear", "Color Box"=14013909}] -> [_ _ w232 _ w260]
          tunnel: w221 -> [_ _ w231 _ w259]
          tunnel: u32[] [15790320, 15790320, 15790320, 15790320, 16777215, 16777215, 15790320, 15790320, 15790320] -> [_ _ _ _ w265]
          tunnel: w219 -> [_ _ _ _ w253]
          tunnel: w216 -> [_ w226 _ _ _]
          frame "Custom", Default {
          }
          frame "Basic" {
            n114 = call <vilib>:"WPI_DashboardUpdateNames.vi"("Controls on Tab"=w226) -> ()  [unwired: 11 in]
          }
          frame "Test" {
            w238 = -2 ("Active Item:Row Number")
            n115 = Index Array(array=w232, index=w231) -> (element=w233:T23)
            n116 = Unbundle(w233) -> ("Operation"=w234:enum16{"Update", "Clear"}, "Color Box"=w235:u32)
            n117 = call <vilib>:"NT Read String.vi"("Name"="TestMode/TestName") -> ("String"=w229:string)  [unwired: 9 in, 1 out]
            n118 = call <vilib>:"NT Read and Format Entries as Tree.vi"("Operation"=w234, "Name Pattern"=w239, "Tree Refnum"=w240) -> ()  [unwired: 7 in, 2 out]
            n119 = case shown="\"\"" w229 {
              tunnel: "TestMode/TestProgress" ("Name") -> [w242 _]
              tunnel: "TestMode/TestProgressText" ("Name") -> [w241 _]
              frame Default {
                n120 = call <vilib>:"NT Read Number.vi"("Name"=w242) -> ("Numeric"=w243:dbl)  [unwired: 9 in, 1 out]
                n121 = call <vilib>:"NT Read String.vi"("Name"=w241) -> ("String"=w244:string)  [unwired: 9 in, 1 out]
                n122 = Bundle("Numeric"=w243, "String"=w244) -> (→"Progress":cluster{"Numeric":dbl, "String":string})  [unwired: 1 in]
              }
              frame "" {
                n123 = property on="Progress" class="Clust (strict)"("Visible"=FALSE) -> ()  [unwired: 2 in, 2 out]
                n124 = local write "Test Name"(u16 0) -> ()
              }
            }
            n125 = property on="Test Tree" class="Tree (strict)"("Active Item Row Number"=w238, "ActiveColNum"=w238, "CellBG"=w235, "Active Item Row Number"=-1 ("Active Item:Row Number"), "CellBG"=u32 5789784 ("Color Box")) -> ()  [unwired: 2 in, 2 out]
          }
          frame "Variables" {
            w250 = string[] ["CameraPublisher", "Usage", "DB"]  # Items to initially close
            n126 = First Call?() -> (First Call?: T/F=w251:bool)
            n127 = control-ref of="Tree"() -> (w252:refnum<vi>)
            n128 = Select(t=w250, s=w251, f=string[] []) -> (s? t:f=w248:string[])
            n129 = call <vilib>:"NT Read and Format Entries as Tree.vi"("Tags to  Close"=w248, "Tree Refnum"=w252) -> ()  [unwired: 8 in, 2 out]
          }
          frame "Commands" {
            w261 = u32 5789784 ("Color Box")
            w262 = T24 {"Row"=-1, "Column"=-2} ("Active Cell:Active Cell")
            w264 = T24 {"Row"=-2, "Column"=-2} ("Active Cell:Active Cell")
            n130 = Index Array(array=w265, index=w259) -> (element=w263:u32)
            n131 = Index Array(array=w260, index=w259) -> (element=w258:T23)
            n132 = Unbundle(w258) -> ("Operation"=w257:enum16{"Update", "Clear"})  [unwired: 1 out]
            n133 = local read "Command Selection"() -> (w256:i32)
            n134 = property on="Command Selection" class="MCListbox (strict)"("ActiveCell"=w264, "CellBG"=w263, "ActiveCell"=w262, "CellBG"=w261) -> ()  [unwired: 2 in, 2 out]
            n135 = call <vilib>:"WPI_DashboardUpdate RPC Info.vi"("Operation"=w257) -> ("update"=w255:bool, "commands"=w254:string[][])  [unwired: 9 in]
            n136 = property on="Command Selection" class="MCListbox (strict)"("ItemNames"=w254) -> ()  [unwired: 2 in, 2 out]
            n137 = property on="Command Params" class="Tbl (strict)"("Active Cell"=w264, "Cell BG Color"=w263, "Active Cell"=w262, "Cell BG Color"=w261) -> ()  [unwired: 2 in, 2 out]
            n138 = call <vilib>:"WPI_DashboardUpdate Command Params.vi"("Update"=w255, "NewVal"=w256, "Commands"=w254, "Param Tbl"=w253) -> ()  [unwired: 7 in, 1 out]
          }
        }
        n139 = call <vilib>:"Connextion Info.vi"() -> ("Connected"=→"NT Connection":bool)  [unwired: 10 in, 1 out]
      }
      event "Test Tree": Value Change {
        # "Show appropriate\ncontrols"
        n140 = event-data() -> ("CtlRef"=w270:refnum<vi>, "NewVal"=w268:string)  [unwired: 1 in]
        n141 = call <vilib>:"WPI_UtilitiesGetTreeIOName.vi"("NewVal"=w268, "TreeControl in"=w270) -> ("I/O Name"=w271:string)  [unwired: 9 in]
        n142 = case shown="\"Camera\"" w271 {
          selector: w271 -> [_ w278 _ w300 w309 _]
          tunnel: w268 -> [_ _ w297 w299 _ w316]
          tunnel: cluster{string[]}[] [{["640x480", "320x240", "160x120"]}, {["Auto", "Fixed indoor", "Fixed outdoor 1", "Fixed outdoor 2", "Fixed fluorescent 1", "Fixed fluorescent 2", "Hold current"]}, {["Auto", "Flicker-free 50 Hz", "Flicker-free 60 Hz", "Hold current"]}, {["None", "Prioritize frame rate", "Prioritize image quality"]}, {["Monochrome", "Color"]}] -> [_ _ _ _ _ w315]
          frame Default {
            w273 = FALSE ("Visible")
            w272 = FALSE ("Visible")
            n143 = property on="Motor" class="Clust (strict)"("Visible"=w272) -> ()  [unwired: 2 in, 2 out]
            n144 = property on="Test Ring" class="Ring (strict)"("Visible"=w272) -> ()  [unwired: 2 in, 2 out]
            n145 = property on="Rev/Fwd" class="Clust (strict)"("Visible"=w273) -> ()  [unwired: 2 in, 2 out]
            n146 = property on="On/Off" class="Bool (strict)"("Visible"=w273) -> ()  [unwired: 2 in, 2 out]
            n147 = property on="Test Slider" class="Slide (strict)"("Visible"=w273) -> ()  [unwired: 2 in, 2 out]
          }
          frame "Analog Out", "Motor", "PWM" {
            w279 = FALSE ("Visible")
            n148 = case shown="\"Analog Out\"" w278 {
              tunnel: [1.0 ("Value") -1.0 ("Value") 0.0 ("Value")] -> w277
              tunnel: [255.0 ("Value") 1.0 ("Value") 5.0 ("Value")] -> w276
              tunnel: [128.0 ("Value") 0.0 ("Value") 0.0 ("Value")] -> w275
              tunnel: [64.0 ("Value") 0.5 ("Value") 1.0 ("Value")] -> w274
              frame "PWM" {
              }
              frame "Motor", Default {
              }
              frame "Analog Out" {
              }
            }
            n149 = property on="Motor" class="Clust (strict)"("Visible"=TRUE) -> ()  [unwired: 2 in, 2 out]
            n150 = property on="Value" class="Slide (strict)"("Value"=w275, "Scale.Minimum"=w277, "Scale.Maximum"=w276, "Scale.Increment"=w274) -> ()  [unwired: 2 in, 2 out]
            n151 = property on="On/Off" class="Bool (strict)"("Visible"=w279) -> ()  [unwired: 2 in, 2 out]
            n152 = property on="Test Slider" class="Slide (strict)"("Visible"=w279) -> ()  [unwired: 2 in, 2 out]
            n153 = property on="Test Ring" class="Ring (strict)"("Visible"=w279) -> ()  [unwired: 2 in, 2 out]
            n154 = property on="Rev/Fwd" class="Clust (strict)"("Visible"=w279) -> ()  [unwired: 2 in, 2 out]
          }
          frame "Servo" {
            w295 = FALSE ("Visible")
            n155 = call <vilib>:"NT Read Number.vi"("Name"=w297) -> ("Numeric"=w296:dbl)  [unwired: 9 in, 1 out]
            n156 = property on="Test Slider" class="Slide (strict)"("Visible"=TRUE, "Scale.Maximum"=170.0 ("Scale.Range:Maximum")) -> ()  [unwired: 2 in, 2 out]
            n157 = local write "Test Slider"(w296) -> ()
            n158 = property on="Motor" class="Clust (strict)"("Visible"=w295) -> ()  [unwired: 2 in, 2 out]
            n159 = property on="Rev/Fwd" class="Clust (strict)"("Visible"=w295) -> ()  [unwired: 2 in, 2 out]
            n160 = property on="On/Off" class="Bool (strict)"("Visible"=w295) -> ()  [unwired: 2 in, 2 out]
            n161 = property on="Test Ring" class="Ring (strict)"("Visible"=w295) -> ()  [unwired: 2 in, 2 out]
          }
          frame "Relay", "Solenoid" {
            w298 = FALSE ("Visible")
            n162 = property on="Motor" class="Clust (strict)"("Visible"=w298) -> ()  [unwired: 2 in, 2 out]
            n163 = property on="Test Slider" class="Slide (strict)"("Visible"=w298) -> ()  [unwired: 2 in, 2 out]
            n164 = Search and Replace String(input string=w299, search string="/Value  **", replace string="/Direction") -> (result string=w305:string)  [unwired: 5 in, 3 out]
            n165 = property on="Test Ring" class="Ring (strict)"("Visible"=w298) -> ()  [unwired: 2 in, 2 out]
            n166 = call <vilib>:"NT Read String.vi"("Name"=w305) -> ("String"=w303:string)  [unwired: 9 in, 1 out]
            n167 = Equal?(x="Both directions", y=w303) -> (x = y?=w301:bool)
            n168 = Not(x=w301) -> (.not. x?=w302:bool)
            n169 = property on="Rev/Fwd" class="Clust (strict)"("Visible"=w301) -> ()  [unwired: 2 in, 2 out]
            n170 = property on="On/Off" class="Bool (strict)"("Visible"=w302, "Caption.Text"=w300) -> ()  [unwired: 2 in, 2 out]
          }
          frame "Compressor", "Digital Out" {
            w308 = FALSE ("Visible")
            # "Get direction and finish"
            n171 = property on="Motor" class="Clust (strict)"("Visible"=w308) -> ()  [unwired: 2 in, 2 out]
            n172 = property on="Test Slider" class="Slide (strict)"("Visible"=w308) -> ()  [unwired: 2 in, 2 out]
            n173 = property on="Test Ring" class="Ring (strict)"("Visible"=w308) -> ()  [unwired: 2 in, 2 out]
            n174 = property on="On/Off" class="Bool (strict)"("Visible"=TRUE, "Caption.Text"=w309) -> ()  [unwired: 2 in, 2 out]
            n175 = property on="Rev/Fwd" class="Clust (strict)"("Visible"=FALSE) -> ()  [unwired: 2 in, 2 out]
          }
          frame "Camera" {
            n176 = call <vilib>:"Get Last Path Segment.vi"("String in"=w316) -> ("String out"=w317:string)  [unwired: 10 in]
            n177 = property on="On/Off" class="Bool (strict)"("Visible"=FALSE) -> ()  [unwired: 2 in, 2 out]
            n178 = property on="Motor" class="Clust (strict)"("Visible"=FALSE) -> ()  [unwired: 2 in, 2 out]
            n179 = property on="Rev/Fwd" class="Clust (strict)"("Visible"=FALSE) -> ()  [unwired: 2 in, 2 out]
            n180 = case shown="\"White Balance  **\"" w317 {
              tunnel: w316 -> [w323 w332 w341 w350 w359 _ w365]
              tunnel: w315 -> [w321 w329 w338 w347 w356 _ _]
              frame "Size  **" {
                n181 = Index Array(array=w321) -> (element=w320:cluster{string[]})  [unwired: 1 in]
                n182 = call <vilib>:"NT Read String.vi"("Name"=w323) -> ("String"=w322:string)  [unwired: 9 in, 1 out]
                n183 = Unbundle(w320) -> (w318:string[])
                n184 = Match First String(2:w318, 3:w322) -> (0:w319:i32)  [unwired: 1 out]
                n185 = property on="Test Ring" class="Ring (strict)"("Value"=w319, "Strings []"=w318) -> ()  [unwired: 2 in, 2 out]
                n186 = property on="Test Ring" class="Ring (strict)"("Visible"=TRUE) -> ()  [unwired: 2 in, 2 out]
                n187 = property on="Test Slider" class="Slide (strict)"("Visible"=FALSE) -> ()  [unwired: 2 in, 2 out]
              }
              frame "White Balance  **" {
                n188 = Index Array(array=w329, index=1) -> (element=w330:cluster{string[]})
                n189 = call <vilib>:"NT Read String.vi"("Name"=w332) -> ("String"=w331:string)  [unwired: 9 in, 1 out]
                n190 = Unbundle(w330) -> (w327:string[])
                n191 = Match First String(2:w327, 3:w331) -> (0:w326:i32)  [unwired: 1 out]
                n192 = property on="Test Ring" class="Ring (strict)"("Value"=w326, "Strings []"=w327) -> ()  [unwired: 2 in, 2 out]
                n193 = property on="Test Ring" class="Ring (strict)"("Visible"=TRUE) -> ()  [unwired: 2 in, 2 out]
                n194 = property on="Test Slider" class="Slide (strict)"("Visible"=FALSE) -> ()  [unwired: 2 in, 2 out]
              }
              frame "Exposure  **" {
                n195 = Index Array(array=w338, index=2) -> (element=w339:cluster{string[]})
                n196 = call <vilib>:"NT Read String.vi"("Name"=w341) -> ("String"=w340:string)  [unwired: 9 in, 1 out]
                n197 = Unbundle(w339) -> (w335:string[])
                n198 = Match First String(2:w335, 3:w340) -> (0:w336:i32)  [unwired: 1 out]
                n199 = property on="Test Ring" class="Ring (strict)"("Value"=w336, "Strings []"=w335) -> ()  [unwired: 2 in, 2 out]
                n200 = property on="Test Ring" class="Ring (strict)"("Visible"=TRUE) -> ()  [unwired: 2 in, 2 out]
                n201 = property on="Test Slider" class="Slide (strict)"("Visible"=FALSE) -> ()  [unwired: 2 in, 2 out]
              }
              frame "Exposure Priority  **" {
                n202 = Index Array(array=w347, index=3) -> (element=w348:cluster{string[]})
                n203 = call <vilib>:"NT Read String.vi"("Name"=w350) -> ("String"=w349:string)  [unwired: 9 in, 1 out]
                n204 = Unbundle(w348) -> (w344:string[])
                n205 = Match First String(2:w344, 3:w349) -> (0:w345:i32)  [unwired: 1 out]
                n206 = property on="Test Ring" class="Ring (strict)"("Value"=w345, "Strings []"=w344) -> ()  [unwired: 2 in, 2 out]
                n207 = property on="Test Ring" class="Ring (strict)"("Visible"=TRUE) -> ()  [unwired: 2 in, 2 out]
                n208 = property on="Test Slider" class="Slide (strict)"("Visible"=FALSE) -> ()  [unwired: 2 in, 2 out]
              }
              frame "Color Enable  **" {
                n209 = Index Array(array=w356, index=4) -> (element=w357:cluster{string[]})
                n210 = call <vilib>:"NT Read String.vi"("Name"=w359) -> ("String"=w358:string)  [unwired: 9 in, 1 out]
                n211 = Unbundle(w357) -> (w353:string[])
                n212 = Match First String(2:w353, 3:w358) -> (0:w354:i32)  [unwired: 1 out]
                n213 = property on="Test Ring" class="Ring (strict)"("Value"=w354, "Strings []"=w353) -> ()  [unwired: 2 in, 2 out]
                n214 = property on="Test Ring" class="Ring (strict)"("Visible"=TRUE) -> ()  [unwired: 2 in, 2 out]
                n215 = property on="Test Slider" class="Slide (strict)"("Visible"=FALSE) -> ()  [unwired: 2 in, 2 out]
              }
              frame Default {
                n216 = property on="Test Ring" class="Ring (strict)"("Visible"=FALSE) -> ()  [unwired: 2 in, 2 out]
                n217 = property on="Test Slider" class="Slide (strict)"("Visible"=FALSE) -> ()  [unwired: 2 in, 2 out]
              }
              frame "Brightness  **", "Color Level  **", "Compression  **", "FPS  **", "Sharpness  **" {
                n218 = call <vilib>:"NT Read Number.vi"("Name"=w365) -> ("Numeric"=w364:dbl)  [unwired: 9 in, 1 out]
                n219 = local write "Test Slider"(w364) -> ()
                n220 = property on="Test Slider" class="Slide (strict)"("Visible"=TRUE, "Scale.Maximum"=100.0 ("Scale.Range:Maximum")) -> ()  [unwired: 2 in, 2 out]
                n221 = property on="Test Ring" class="Ring (strict)"("Visible"=FALSE) -> ()  [unwired: 2 in, 2 out]
              }
            }
          }
        }
        n222 = property on="Progress" class="Clust (strict)"("Visible"=FALSE) -> ()  [unwired: 2 in, 2 out]
      }
      event "Test Name": Mouse Enter {
        # "Populate the ring with the list of tests"
        n223 = event-data() -> ()  [unwired: 1 in, 1 out]
        n224 = call <vilib>:"NT Read String Array.vi"("Name"="TestMode/TestList") -> ("String Array"=w373:string[])  [unwired: 9 in, 1 out]
        n225 = Build Array (concatenate)("Select the test to run...", w373) -> (w372:string[])
        n226 = property on="Test Name" class="Ring (strict)"("Strings []"=w372) -> ()  [unwired: 2 in, 2 out]
      }
      event "Test Name": Value Change {
        w375 = FALSE ("Visible")
        # "Tell the robot the test name to run"
        n227 = event-data() -> ("NewVal"=w379:u16)  [unwired: 1 in]
        n228 = property on="Test Name" class="Ring (strict)"() -> ("Strings []"=w380:string[])  [unwired: 2 in, 2 out]
        n229 = local write "Progress"(T6 {"Test Progress"=0, "Test Progress Text"=""} ("Progress")) -> ()
        n230 = Index Array(array=w380, index=w379) -> (element=w378:string)
        n231 = call <vilib>:"NT Write String.vi"("String"=w378, "Name"="TestMode/TestName") -> ()  [unwired: 9 in, 1 out]
        n232 = property on="Progress" class="Clust (strict)"("Visible"=TRUE) -> ()  [unwired: 2 in, 2 out]
        n233 = property on="Motor" class="Clust (strict)"("Visible"=w375) -> ()  [unwired: 2 in, 2 out]
        n234 = property on="Test Slider" class="Slide (strict)"("Visible"=w375) -> ()  [unwired: 2 in, 2 out]
        n235 = property on="On/Off" class="Bool (strict)"("Visible"=w375) -> ()  [unwired: 2 in, 2 out]
        n236 = property on="Rev/Fwd" class="Clust (strict)"("Visible"=w375) -> ()  [unwired: 2 in, 2 out]
        n237 = property on="Test Ring" class="Ring (strict)"("Visible"=w375) -> ()  [unwired: 2 in, 2 out]
      }
      event "Select Auto": Mouse Enter {
        # "Populate the combo box with the list of autonomous options"
        n238 = event-data() -> ()  [unwired: 1 in, 1 out]
        n239 = call <vilib>:"NT Read String Array.vi"("Name"="Auto List") -> ("String Array"=w382:string[])  [unwired: 9 in, 1 out]
        n240 = property on="Select Auto" class="CmbBox"("Strings[]"=w382) -> ()  [unwired: 2 in, 2 out]
      }
      event "Select Auto": Value Change {
        # "User modified the Auto Selection. Write to NT variable so robot knows."
        n241 = event-data() -> ("NewVal"=w385:string)  [unwired: 1 in]
        n242 = call <vilib>:"NT Write String.vi"("String"=w385, "Name"="Auto Selector") -> ()  [unwired: 9 in, 1 out]
      }
      event "Command Selection": Value Change {
        # "Get the params and show in table"
        n243 = event-data() -> ("NewVal"=w391:i32)  [unwired: 1 in]
        n244 = property on="Command Selection" class="MCListbox (strict)"() -> ("ItemNames"=w389:string[][])  [unwired: 2 in, 2 out]
        n245 = call <vilib>:"WPI_DashboardUpdate Command Params.vi"("NewVal"=w391, "Commands"=w389, "Param Tbl"=w390) -> ()  [unwired: 8 in, 1 out]
      }
      event "Execute Command": Value Change {
        # "Started one, Unique ID holds\nresponse"
        n246 = event-data() -> ()  [unwired: 1 in, 1 out]
        n247 = property on="Command Selection" class="MCListbox (strict)"() -> ("ItemNames"=w402:string[][])  [unwired: 2 in, 2 out]
        n248 = Index Array(array=w402, index (row)="Command Selection", index (col)=0) -> (element=w400:string)
        n249 = call <vilib>:"Invoke Commands.vi"("Command Params"="Command Params", "Function Name"=w400) -> ("Params"=w396:u8, "Started"=w395:bool)  [unwired: 7 in, 1 out]
        n250 = Array Subset(array="Command Params", length (row)=w396) -> (w397:string[][])  [unwired: 3 in]
        n251 = Select(t="Executing" ("Cmd Status"), s=w395, f="" ("Cmd Status")) -> (s? t:f=→"Cmd Status":string)
      }
      event "Command Selection": Double Click {
        n252 = event-data() -> ("Row"=w410:i32)  [unwired: 1 in]
        n253 = property on="Command Selection" class="MCListbox (strict)"() -> ("ItemNames"=w413:string[][])  [unwired: 2 in, 2 out]
        n254 = local read "Command Params"() -> (w409:string[][])
        n255 = Index Array(array=w413, index (row)=w410, index (col)=0) -> (element=w411:string)
        n256 = call <vilib>:"Invoke Commands.vi"("Command Params"=w409, "Function Name"=w411) -> ("Params"=w408:u8, "Started"=w403:bool)  [unwired: 7 in, 1 out]
        n257 = Array Subset(array=w409, length (row)=w408) -> (w407:string[][])  [unwired: 3 in]
        n258 = Select(t="Executing" ("Cmd Status"), s=w403, f="" ("Cmd Status")) -> (s? t:f=w404:string)
        n259 = local write "Cmd Status"(w404) -> ()
      }
      event "CheckList": Double Click {
        # "Shift clears all"
        # "Update symbols on the listbox"
        n260 = event-data() -> ("PlatMods.Shift"=w415:bool, "Row"=w417:i32)  [unwired: 1 in]
        n261 = case shown="True" w415 {
          tunnel: w417 -> [w421 _]
          tunnel: 1 -> [w420 _]
          frame False {
            n262 = property on="CheckList" class="LstBox (strict)"() -> ("Item Symbols"=w419:i32[])  [unwired: 2 in, 2 out]
            n263 = Replace Array Subset(array=w419, new element=w420, index=w421) -> (w418:i32[])
            n264 = property on="CheckList" class="LstBox (strict)"("Item Symbols"=w418) -> ()  [unwired: 2 in, 2 out]
          }
          frame True {
            w422 = 0 ("Top Row")
            n265 = property on="CheckList" class="LstBox (strict)"() -> ("Number of Rows"=w424:u32)  [unwired: 2 in, 2 out]
            n266 = Initialize Array(0, w424) -> (w423:i32[])
            n267 = property on="CheckList" class="LstBox (strict)"("Top Row"=w422, "Value"=w422, "Item Symbols"=w423) -> ()  [unwired: 2 in, 2 out]
          }
        }
      }
      event "CheckList": Key Down {
        # "Update symbols on the listbox\nLeft and right keys check and uncheck"
        n268 = event-data() -> ("VKey"=w428:T21)  [unwired: 1 in]
        n269 = case shown="\"Left\", \"Right\"" w428 {
          selector: w428 -> [w433 _]
          tunnel: eventvkey."Left" ("VKey") -> [w431 _]
          frame "Left", "Right" {
            n270 = Equal?(x=w431, y=w433) -> (x = y?=w432:bool)
            n271 = Select(t=0, s=w432, f=1) -> (s? t:f=w434:i32)
            n272 = property on="CheckList" class="LstBox (strict)"() -> ("Item Symbols"=w437:i32[])  [unwired: 2 in, 2 out]
            n273 = Replace Array Subset(array=w437, new element=w434, index="CheckList") -> (w436:i32[])
            n274 = property on="CheckList" class="LstBox (strict)"("Item Symbols"=w436) -> ()  [unwired: 2 in, 2 out]
          }
          frame Default {
          }
        }
      }
      event "Motor.Enable": Value Change {
        # "When the test mode otor enable helper is set, update that\ntree row item's value"
        n275 = event-data() -> ("NewVal"=w443:bool)  [unwired: 1 in]
        n276 = Unbundle("Motor") -> ("Value"=w442:dbl)  [unwired: 1 out]
        n277 = Select(t=w442, s=w443, f=0.0) -> (s? t:f=w440:dbl)
        n278 = call <vilib>:"NT Write Number.vi"("Numeric"=w440, "Name"=w439) -> ()  [unwired: 9 in, 1 out]
      }
      event "Test Slider": Value Change {
        # "When the test mode slider helper is set, update that\ntree row item's value"
        n279 = event-data() -> ("NewVal"=w446:dbl)  [unwired: 1 in]
        n280 = call <vilib>:"NT Write Number.vi"("Numeric"=w446, "Name"=w447) -> ()  [unwired: 9 in, 1 out]
      }
      event "On/Off": Value Change {
        # "When the test mode on/off helper value is set, update that\ntree row item's value"
        n281 = event-data() -> ("NewVal"=w451:bool)  [unwired: 1 in]
        n282 = Boolean To (0,1)(Boolean=w451) -> (0, 1=w450:i16)
        n283 = call <vilib>:"NT Write Number.vi"("Numeric"=w450, "Name"=w449) -> ()  [unwired: 9 in, 1 out]
      }
      event "Rev/Fwd": Value Change {
        # "When the test mode helper value for relays is set, update that\ntree row item's value"
        n284 = event-data() -> ("NewVal.Forward"=w459:bool, "NewVal.Reverse"=w458:bool)  [unwired: 1 in]
        n285 = Boolean To (0,1)(Boolean=w459) -> (0, 1=w455:i16)
        n286 = Boolean To (0,1)(Boolean=w458) -> (0, 1=w457:i16)
        n287 = Negate(x=w457) -> (-x=w456:i16)
        n288 = Add(x=w455, y=w456) -> (x+y=w454:i16)
        n289 = call <vilib>:"NT Write Number.vi"("Numeric"=w454, "Name"=w453) -> ()  [unwired: 9 in, 1 out]
      }
      event "Test Ring": Value Change {
        # "When a test mode helper value is selected from the ring,\nset the tree item's variable to the string value"
        n290 = event-data() -> ("NewVal"=w463:u16)  [unwired: 1 in]
        n291 = property on="Test Ring" class="Ring (strict)"() -> ("Strings []"=w464:string[])  [unwired: 2 in, 2 out]
        n292 = Index Array(array=w464, index=w463) -> (element=w462:string)
        n293 = call <vilib>:"NT Write String.vi"("String"=w462, "Name"=w461) -> ()  [unwired: 9 in, 1 out]
      }
      event "Rec Mode": Value Change {
        # "Update globals for recording mode and path to read log from.\nClear when logging and let NetworkTables set path for vision to\nuse."
        n294 = event-data() -> ("NewVal"=w475:enum32{"Stop", "Record", "Playback"})  [unwired: 1 in]
        n295 = global write "WPI_DashboardLogging Global.vi" "Logging Filename"(path "") -> ()
        n296 = global write "WPI_DashboardLogging Global.vi" "Recording"(w475) -> ()
        n297 = case shown="\"Playback\"" w475 {
          tunnel: w474 -> [_ w477 w486]
          tunnel: [_ _ w485] -> w472
          tunnel: [_ _ w484] -> _
          tunnel: w470 -> [_ _ w482]
          tunnel: cluster{i32, i32} {-250, 170} -> [_ _ w481]
          tunnel: [_ _ T22 {"Image Size"=TRUE, "Image Type"=TRUE, "Pixel Value"=TRUE, "ROI Information"=TRUE, "Zoom Factor"=FALSE} ("Image Information Shown:All Elements")] -> w465
          tunnel: [_ _ TRUE ("Zoom Factor")] -> w466
          tunnel: w468 -> [_ _ w478]
          frame Default {
          }
          frame "Stop", "Record" {
            # "Place Window too"
            n298 = invoke class="VI" method="FP.Close"(reference=w477) -> (reference out=w476:refnum<vi>)  [unwired: 2 in, 2 out]
            n299 = invoke class="VI" method="Abort VI"(reference=w476) -> ()  [unwired: 2 in, 3 out]
          }
          frame "Playback" {
            n300 = call "Open Playback Panel.vi"("Offset"=w481, "DB VI Ref"=w482, "Playback in"=w486) -> ("Playback out"=w483:refnum<vi>)  [unwired: 8 in]
            n301 = register-events(w483, w478) -> (reference out=w485:refnum<event-registration>, error out=w484:errorcluster)  [unwired: 2 in]
          }
        }
        n302 = property on="Camera Image Right" class="ImageControl"("Image Information Shown"=w465, "Image Information Visible"=w466) -> ()  [unwired: 2 in, 2 out]
        n303 = property on="Camera Image" class="ImageControl"("Image Information Shown"=w465, "Image Information Visible"=w466) -> ()  [unwired: 2 in, 2 out]
        n304 = call <vilib>:"WPI_DashboardNT Log FieldName Cache.vi"("Operation"=enum16{"Lookup/Add", "Index", "Clear"}."Clear") -> ()  [unwired: 8 in, 3 out]
      }
      event Panel Close {
        w488 = enum32{"Stop", "Record", "Playback"}."Stop" ("Rec Mode")
        # "Playback window has been closed, abort"
        n305 = event-data() -> ()  [unwired: 1 in, 4 out]
        n306 = local write "Rec Mode"(w488) -> ()
        n307 = global write "WPI_DashboardLogging Global.vi" "Recording"(w488) -> ()
      }
      event Panel Close {
        # "Abort playback window and ourself"
        n308 = event-data() -> ()  [unwired: 1 in, 4 out]
        n309 = invoke class="VI" method="FP.Close"(reference=w492) -> (reference out=w491:refnum<vi>)  [unwired: 2 in, 2 out]
        n310 = invoke class="VI" method="Abort VI"(reference=w491) -> (error out=w490:errorcluster)  [unwired: 2 in, 2 out]
        n311 = invoke class="VI" method="Abort VI"(error in=w490) -> ()  [unwired: 2 in, 3 out]
      }
      event User Event {
        n312 = event-data() -> ("IDs"=w499:cluster{"RPC field ID":u16, "Unique ID":u16}, "String"=w498:string)  [unwired: 1 in]
        n313 = Bundle("IDs"=w499, "String"=w498) -> (w497:T9)  [unwired: 1 in]
        n314 = call <vilib>:"Retrieve RPC Response.vi"("RPC Response"=w497) -> ("Output"=w495:string[][])  [unwired: 10 in]
        n315 = Build Array (concatenate)(w493, w495) -> (w494:string[][])
        n316 = local write "Command Params"(w494) -> ()
        n317 = local write "Cmd Status"("" ("Cmd Status")) -> ()
      }
      event "Tree": Double Click {
        n318 = event-data() -> ("PlatMods"=w505:T25, "Tag"=w502:string)  [unwired: 1 in]
        n319 = Unbundle(w505) -> ("Shift"=w504:bool)  [unwired: 4 out]
        n320 = String Subset(string=w502, length (rest)=1 ("length (rest)")) -> (substring=w501:string)  [unwired: 1 in]
        n321 = Not(x=w504) -> (.not. x?=w503:bool)
        n322 = case shown="\"/\"" w501 {
          tunnel: w502 -> [_ w508]
          tunnel: w503 -> [_ w507]
          frame Default {
          }
          frame "/" {
            n323 = call <vilib>:"NT Update Persistence.vi"("Persistence"=w507, "Name"=w508) -> ()  [unwired: 9 in, 1 out]
          }
        }
      }
    }
  }
  n324 = while {
    tunnel: w65 -> [w510]
    i -> [w513]
    stop <- FALSE stop-if-true
    n325 = Wait (ms)(milliseconds to wait=u32 100) -> ()  [unwired: 1 out]
    n326 = case shown="\"Playback\"" "Rec Mode" {
      tunnel: w513 -> [_ _ w528]
      tunnel: [u32 2829099 ("Base Color") u32 11141120 ("Target Color") w517] -> w509
      frame "Stop", Default {
        # "Reset the color, extra updates don't cost much"
      }
      frame "Record" {
      }
      frame "Playback" {
        # "Playback"
        n327 = Quotient & Remainder(x=w528, y=u32 50 ("milliseconds to wait")) -> (x-y*floor(x/y)=w524:u32)  [unwired: 1 out]
        n328 = Divide(x=w524, y=u32 50 ("milliseconds to wait")) -> (x/y=w521:dbl)
        n329 = Multiply(x=6.283185307179586, y=w521) -> (x*y=w526:dbl)
        n330 = Sine(x=w526) -> (sin(x)=w525:dbl)
        n331 = Absolute Value(x=w525) -> (abs(x)=w518:dbl)
        n332 = call "Interpolate RGB Color.vi"("Proportion"=w518, "Target Color"=u32 30976, "Base Color"=u32 2829099) -> ("Result Color"=w517:u32)  [unwired: 8 in]
      }
    }
    n333 = property class="Pane"(reference=w510, "PaneColor"=w509) -> ()  [unwired: 1 in, 2 out]
  }
  n334 = local write "Dashboard Tab"(T2."Drive" ("Dashboard Tab")) -> ()
  n335 = property on="On/Off" class="Bool (strict)"("Visible"=w36) -> ()  [unwired: 2 in, 2 out]
  n336 = property on="Motor" class="Clust (strict)"("Visible"=w36) -> ()  [unwired: 2 in, 2 out]
  n337 = property on="Progress" class="Clust (strict)"("Visible"=w36) -> ()  [unwired: 2 in, 2 out]
  n338 = property on="Test Ring" class="Ring (strict)"("Visible"=w36) -> ()  [unwired: 2 in, 2 out]
  n339 = property on="Rev/Fwd" class="Clust (strict)"("Visible"=w36) -> ()  [unwired: 2 in, 2 out]
  n340 = while {
    tunnel: u16 1741 ("timeout ms (25000)") -> [w530]
    stop <- FALSE stop-if-true
    n341 = TCP Create Listener(10:w530) -> (0:w529:errorcluster, 3:w531:refnum<k5>)  [unwired: 4 in, 1 out]
    n342 = case shown="No Error" w529 {
      selector: w529 -> [w533 _]
      tunnel: w531 -> [w534 _]
      frame No Error {
        n343 = while {
          tunnel: w534 -> [w537]
          tunnel: w533 -> [w536]
          stop <- FALSE stop-if-true
          n344 = TCP Wait On Listener(8:w536, 11:w537) -> (0:w538:errorcluster, 4:w539:refnum<k5>)  [unwired: 2 in, 3 out]
          n345 = local write "TCP"(w539) -> ()
          n346 = case shown="No Error" w538 {
            frame No Error {
            }
            frame Error {
              n347 = Wait (ms)(milliseconds to wait=u32 1000) -> ()  [unwired: 1 out]
            }
          }
        }
      }
      frame Error {
        n348 = Wait (ms)(milliseconds to wait=u32 1000) -> ()  [unwired: 1 out]
      }
    }
  }
  n349 = local write "Command Selection"(u16 0 ("milliseconds to wait")) -> ()
  n350 = local write "Command Params"(string[][] [] ("Command Params")) -> ()
  n351 = global write "WPI_DashboardLogging Global.vi" "Recording"(w59) -> ()
  n352 = local write "Rec Mode"(w59) -> ()
  n353 = call <vilib>:"NT Write String.vi"("String"="Select Auto", "Name"="Auto Selector") -> ()  [unwired: 9 in, 1 out]
